vi "Task.vi"(8 "error in (no error)":errorcluster, 10 "Mixer":dbl(ring) items=["0%"=0.075, "25%"=0.08, "50%"=0.085, "75%"=0.09, "100%"=0.095], 11 "Feeder in":refnum<class "Feeder.lvclass">) -> (0 "error out":errorcluster, 3 "Feeder out":refnum<class "Feeder.lvclass">)   [LabVIEW 2018, in "Feeder Actor.lvlib" / "Feeder.lvclass"]
uses:
  Feeder.lvclass
  <vilib>/ActorFramework/Actor/Actor.lvclass
  C:/Program Files/National Instruments/LabVIEW 2018/vi.lib/ActorFramework/Actor/Actor.lvclass
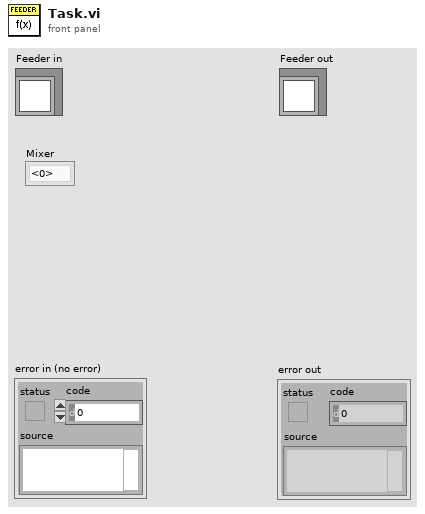
[diagram p1: front panel]
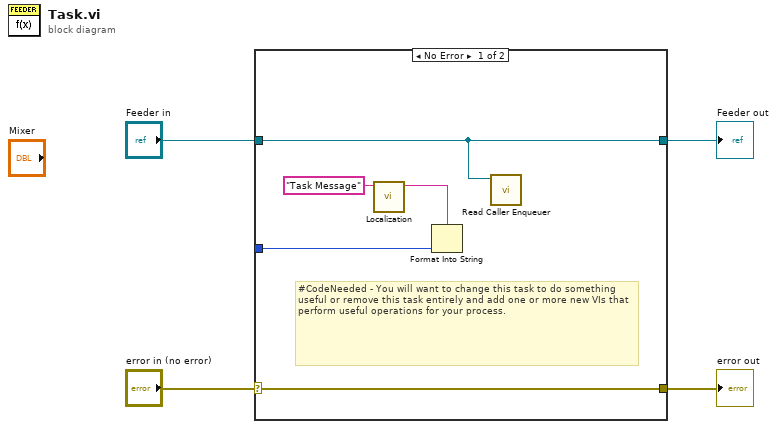
[diagram p0: block diagram]
diagram:
  n1 = case shown="No Error" "error in (no error)" {
    selector: "error in (no error)" -> [w10 w12]
    tunnel: [w10 w12] -> w4
    tunnel: [w9 w11] -> w2
    tunnel: "Feeder in" -> [w9 w11]
    tunnel: [w6 _] -> w1
    frame No Error {
      # "#CodeNeeded - You will want to change this task to do something useful or remove this task entirely and add one or more new VIs that perform useful operations for your process."
      n2 = call "Localization.vi"("Unlocalized"="Task Message") -> ("Localized"=w7:string)  [unwired: 10 in]
      n3 = Format Into String(format string=w7, w6) -> ()  [unwired: 2 in, 2 out]
      n4 = call <vilib>:"Read Caller Enqueuer.vi"("Actor"=w9) -> ()  [unwired: 10 in, 1 out]
    }
    frame Error {
    }
  }
  "error out" <- w4
  "Feeder out" <- w2
